vi "RP convert raw data.vi"(7 "Max Volts":sgl[](array[numeric])=[20.0, 1.0], 8 "Error In":errorcluster, 10 "Format":T1=enum."Digitizer", 11 "data stream":string) -> (0 "Error Out":errorcluster, 1 "element":u32, 2 "phase out":u32[](array[numeric]), 3 "data out":sgl[][](array[numeric]))   [LabVIEW 2015]
uses:
  Mode.ctl
  RP ADC to Volts 1D.vi
  RP 32 ADC to Volts 1D.vi
  RP ADC to Volts 2D.vi
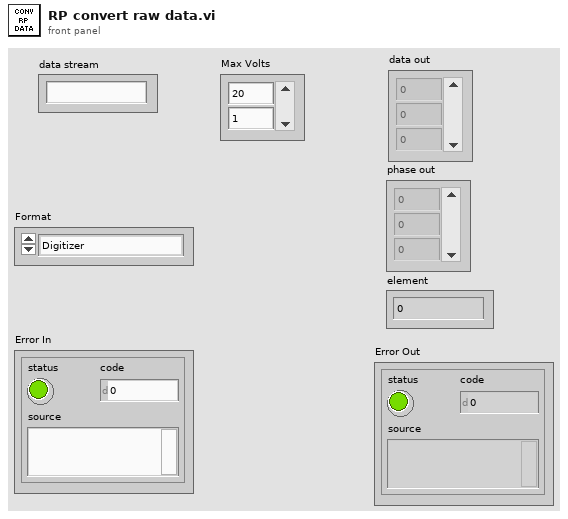
[diagram p1: front panel]
types:
  T1 = typedef "Mode.ctl" = enum16{"Filter", "Lockin test", "Snapshot test", "Digitizer"}
  T2 = enum16{"big-endian, network order", "native, host order", "little-endian"}
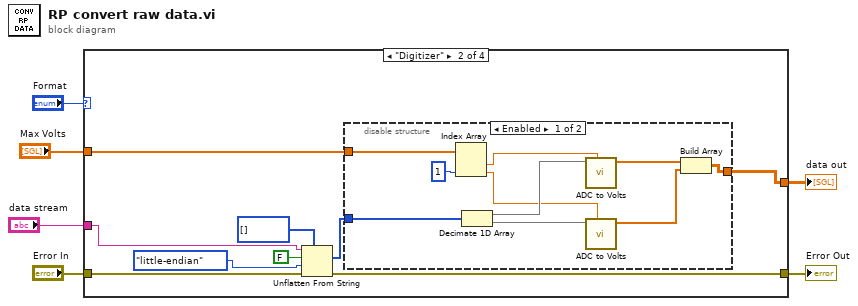
[diagram p0: block diagram]
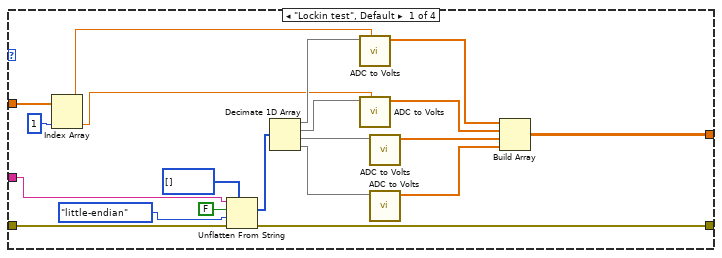
[diagram p2: hidden frame]
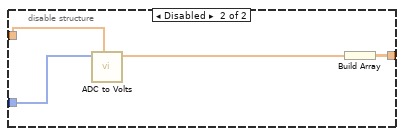
[diagram p3: hidden frame]
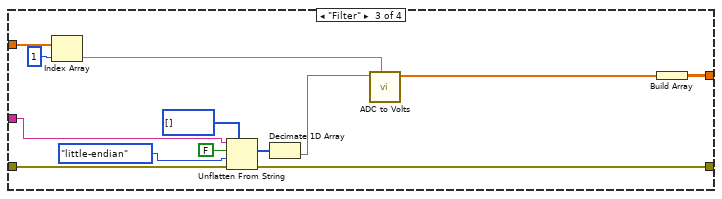
[diagram p4: hidden frame]
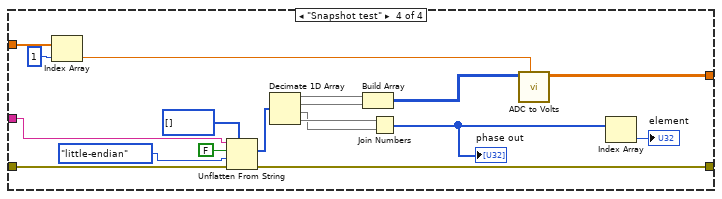
[diagram p5: hidden frame]
diagram:
  n1 = case shown="\"Digitizer\"" "Format" {
    tunnel: [w26 w28 w62 w75] -> w4
    tunnel: "Max Volts" -> [w17 w29 w59 w74]
    tunnel: "data stream" -> [w11 w33 w56 w70]
    tunnel: "Error In" -> [w12 w32 w55 w68]
    tunnel: [w10 w27 w52 w67] -> w1
    frame "Lockin test", Default {
      n2 = Index Array(array=w17, index #2=1 ("index")) -> (element #1=w9:sgl, element #2=w8:sgl)  [unwired: 1 in]
      n3 = Unflatten From String(type=i16[] [], binary string=w11, data includes array or string size? (T)=FALSE, byte order (0:big-endian, network order)=T2."little-endian", error in (no error)=w12) -> (value=w13:i16[], error out=w10:errorcluster)  [unwired: 1 out]
      n4 = Decimate 1D Array(w13) -> (w25:i16[], w23:i16[], w21:i16[], w20:i16[])
      n5 = call-poly "ADC to Volts.vi"("Max Volts"=w9, "ADC data"=w25) -> ("Volts"=w24:sgl[])  [unwired: 9 in]
      n6 = call-poly "ADC to Volts.vi"("Max Volts"=w8, "ADC data"=w23) -> ("Volts"=w22:sgl[])  [unwired: 9 in]
      n7 = call-poly "ADC to Volts.vi"("ADC data"=w21) -> ("Volts"=w18:sgl[])  [unwired: 10 in]
      n8 = call-poly "ADC to Volts.vi"("ADC data"=w20) -> ("Volts"=w19:sgl[])  [unwired: 10 in]
      n9 = Build Array(w24, w22, w18, w19) -> (w26:sgl[][])
    }
    frame "Digitizer" {
      n10 = Unflatten From String(type=i16[] [], binary string=w33, data includes array or string size? (T)=FALSE, byte order (0:big-endian, network order)=T2."little-endian", error in (no error)=w32) -> (value=w30:i16[], error out=w27:errorcluster)  [unwired: 1 out]
      n11 = disable-structure shown="Enabled" {
        disable-tunnel: [w40 w46] -> w28
        disable-tunnel: w30 -> [w45 w48]
        disable-tunnel: w29 -> [w38 w49]
        frame Enabled {
          n12 = Index Array(array=w38, index #2=1 ("index")) -> (element #1=w36:sgl, element #2=w37:sgl)  [unwired: 1 in]
          n13 = Decimate 1D Array(w45) -> (w44:i16[], w43:i16[])
          n14 = call-poly "ADC to Volts.vi"("Max Volts"=w36, "ADC data"=w44) -> ("Volts"=w42:sgl[])  [unwired: 9 in]
          n15 = call-poly "ADC to Volts.vi"("Max Volts"=w37, "ADC data"=w43) -> ("Volts"=w41:sgl[])  [unwired: 9 in]
          n16 = Build Array(w42, w41) -> (w40:sgl[][])
        }
        frame Disabled {
          n17 = call-poly "ADC to Volts.vi"("Max Volts"=w49, "ADC data"=w48) -> ("Volts"=w47:sgl[])  [unwired: 9 in]
          n18 = Build Array(w47) -> (w46:sgl[][])
        }
      }
    }
    frame "Filter" {
      n19 = Index Array(array=w59, index=1) -> (element=w51:sgl)
      n20 = Unflatten From String(type=i32[] [], binary string=w56, data includes array or string size? (T)=FALSE, byte order (0:big-endian, network order)=T2."little-endian", error in (no error)=w55) -> (value=w53:i32[], error out=w52:errorcluster)  [unwired: 1 out]
      n21 = Decimate 1D Array(w53) -> (w61:i32[])  [unwired: 1 out]
      n22 = call-poly "ADC to Volts.vi"("Max Volts"=w51, "ADC data"=w61) -> ("Volts"=w60:sgl[])  [unwired: 9 in]
      n23 = Build Array(w60) -> (w62:sgl[][])
    }
    frame "Snapshot test" {
      n24 = Index Array(array=w74, index=1) -> (element=w66:sgl)
      n25 = Unflatten From String(type=i16[] [], binary string=w70, data includes array or string size? (T)=FALSE, byte order (0:big-endian, network order)=T2."little-endian", error in (no error)=w68) -> (value=w69:i16[], error out=w67:errorcluster)  [unwired: 1 out]
      n26 = Decimate 1D Array(w69) -> (w80:i16[], w79:i16[], w77:i16[], w78:i16[])
      n27 = Build Array(w80, w79) -> (w76:i16[][])
      n28 = Join Numbers(hi=w78, lo=w77) -> ((hi.lo)=w64:u32[])
      "phase out" <- w64
      n29 = call-poly "ADC to Volts.vi"("Max Volts"=w66, "ADC data"=w76) -> ("Volts"=w75:sgl[][])  [unwired: 9 in]
      n30 = Index Array(array=w64) -> (element=→"element":u32)  [unwired: 1 in]
    }
  }
  "Error Out" <- w1
  "data out" <- w4
